vi "call a simple cuda cll.vi"() -> ()   [LabVIEW 2017]
uses:
  D:/Documents/Visual Studio 2015/Projects/CudaDll32/x64/Release/CudaDll32.dll
panel:
  out "a":i32[](array[numeric])
  out "c":i32[](array[numeric])
  in  "Numeric":i32
  in  "Array out":i32[](array[numeric])
  in  "Array 2":i32[](array[numeric])
  in  "Array":i32[](array[numeric])
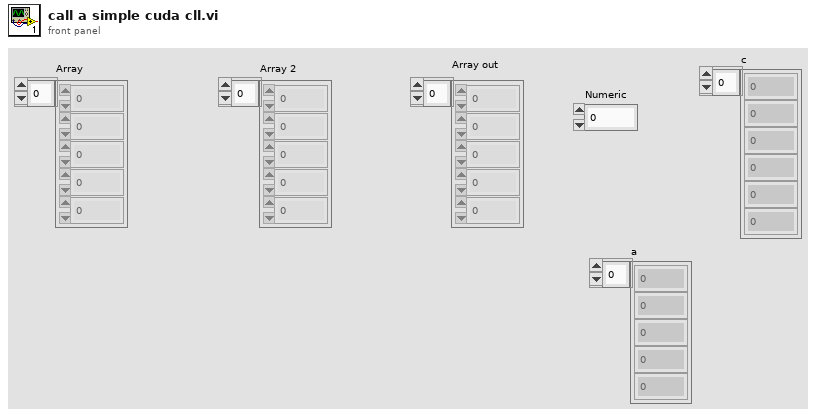
[diagram p1: front panel]
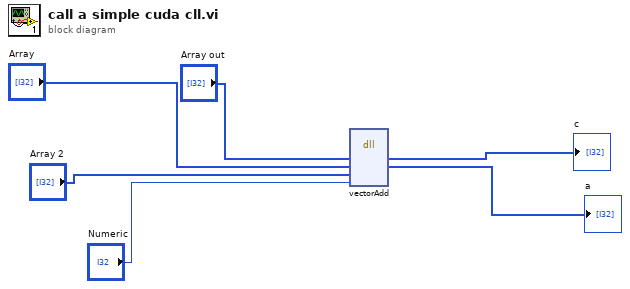
[diagram p0: block diagram]
diagram:
  n1 = dll-call lib="D:/Documents/Visual Studio 2015/Projects/CudaDll32/x64/Release/CudaDll32.dll" fn="vectorAdd"("c"="Array out", "a"="Array", "b"="Array 2", "size"="Numeric") -> ("c"=→"c":i32[], "a"=→"a":i32[])  [unwired: 6 in, 2 out]
